vi "Add Bitfile Dependency.vi"(8 "error in (no error)":errorcluster, 10 "Path":path, 11 "Item Ref in":T1 format="%.0x") -> (0 "error out":errorcluster, 3 "Item Ref out":T1 format="%.0x")   [LabVIEW 2018, in "FPGA Addon System Explorer.lvlib"]
uses:
  FPGA Addon System Explorer.lvlib
  <vilib>/NI Veristand/Custom Device API/Custom Device Item Ref.ctl
  <vilib>/NI Veristand/Custom Device API/Dependent File Optional Info.ctl
  Addon Shared/SubVIs/Constants.vi
  <vilib>/NI Veristand/Custom Device API/Set Item Property (Dependent File).vi
  <vilib>/NI Veristand/Custom Device API/Custom Device API.lvlib
  Addon Shared/FPGA Addon Shared.lvlib
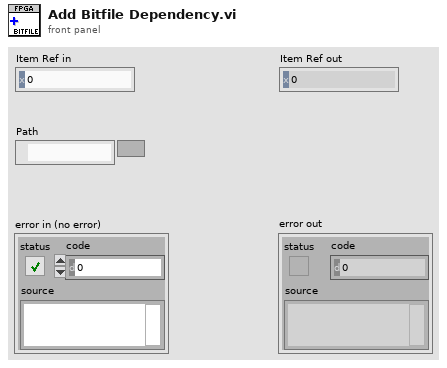
[diagram p1: front panel]
types:
  T1 = typedef "Custom Device API.lvlib/Custom Device Item Ref.ctl" = u64
  T2 = typedef "Custom Device API.lvlib/Dependent File Optional Info.ctl" = cluster{"Version":string, "RTDestination":path, "ForceDownload":bool, "SupportedTarget":string, "MD5":string}
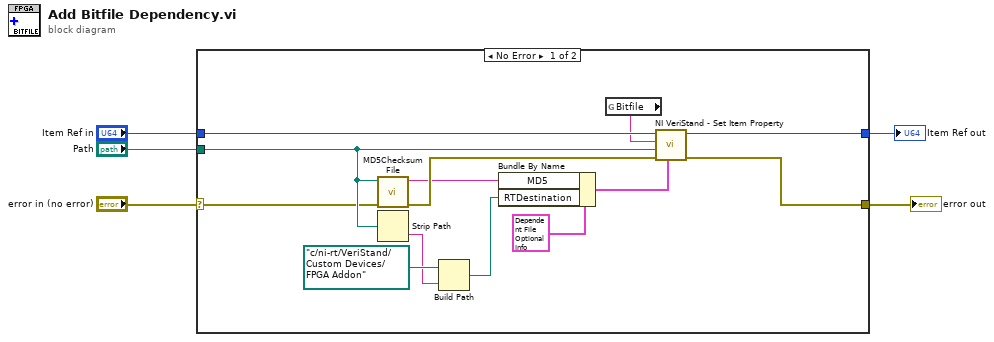
[diagram p0: block diagram]
diagram:
  n1 = case shown="No Error" "error in (no error)" {
    selector: "error in (no error)" -> [w6 w20]
    tunnel: "Item Ref in" -> [w18 w19]
    tunnel: [w13 w20] -> w4
    tunnel: [w12 w19] -> w3
    tunnel: "Path" -> [w10 _]
    frame No Error {
      n2 = call <vilib>:"MD5Checksum File.vi"("error in (no error)"=w6, "Path"=w10) -> ("error out"=w17:errorcluster, "MD5 message-digest"=w16:string)  [unwired: 8 in]
      n3 = Strip Path(path=w10) -> (name=w8:string)  [unwired: 1 out]
      n4 = Build Path(base path=path "c:/ni-rt/VeriStand/Custom Devices/FPGA Addon" ("RTDestination"), name or relative path=w8) -> (appended path=w7:path)
      n5 = Bundle By Name(cluster=T2 {"Version"="1.0", "RTDestination"=path "c:/ni-rt/VeriStand/Custom Devices/FPGA Addon", "ForceDownload"=FALSE, "SupportedTarget"="All", "MD5"=""} ("OptionalInfo"), "MD5"=w16, "RTDestination"=w7) -> (w15:T2)
      n6 = global read "Constants.vi" "Bitfile"() -> (w11:string)
      n7 = call-poly <vilib>:"NI VeriStand - Set Item Property.vi"("OptionalInfo"=w15, "error in (no error)"=w17, "Path"=w10, "Property Name"=w11, "Item Ref in"=w18) -> ("error out"=w13:errorcluster, "Item Ref out"=w12:T1)  [unwired: 4 in, 1 out]
    }
    frame Error {
    }
  }
  "error out" <- w4
  "Item Ref out" <- w3
